vi "Antenna Comms.vi"() -> ()   [LabVIEW 2019]
panel:
  out "state":enum16{"connect", "run", "close"}(ring)
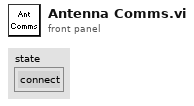
[diagram p1: front panel]
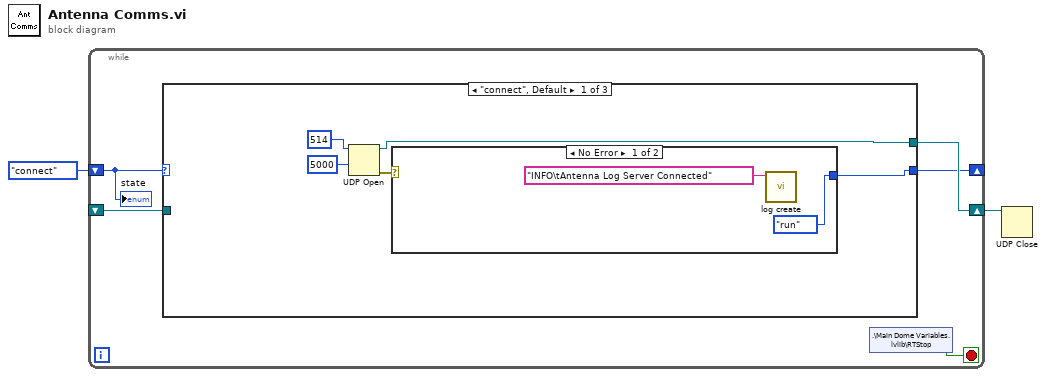
[diagram p0: block diagram]
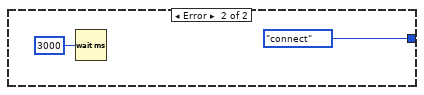
[diagram p2: hidden frame]
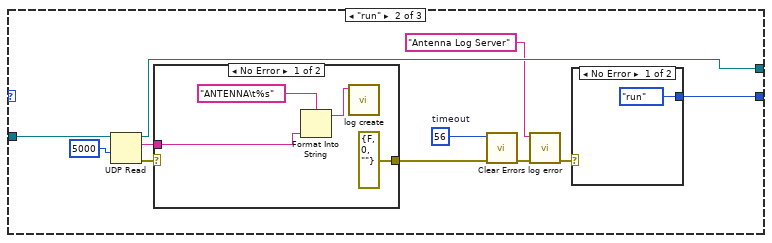
[diagram p3: hidden frame]
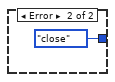
[diagram p4: hidden frame]
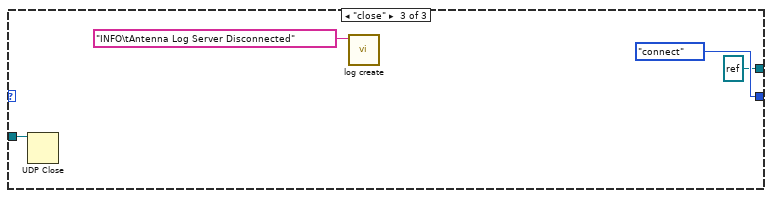
[diagram p6: hidden frame]
diagram:
  n1 = while {
    shift-right: [w3] -> _
    shift-left: enum16{"connect", "run", "close"}."connect" ("y") -> [w6]
    shift-right: [w5] -> w1
    shift-left: _ -> [w4]
    stop <- w7 stop-if-true
    n2 = case shown="\"connect\", Default" w6 {
      tunnel: [w10 w20 refnum<k16> refnum ("port")] -> w5
      tunnel: w4 -> [_ w27 w36]
      tunnel: [w8 w23 enum16{"connect", "run", "close"}."connect" ("y")] -> w3
      frame "connect", Default {
        n3 = UDP Open(9:5000 ("timeout ms (25000)"), 11:u16 514 ("port")) -> (port=w10:refnum<k16>, 0:w9:errorcluster)  [unwired: 3 in, 1 out]
        n4 = case shown="No Error" w9 {
          tunnel: [enum16{"connect", "run", "close"}."run" ("y") enum16{"connect", "run", "close"}."connect" ("y")] -> w8
          frame No Error {
            n5 = call "log create.vi"("message"="INFO\tAntenna Log Server Connected") -> ()  [unwired: 11 in]
          }
          frame Error {
            n6 = Wait (ms)(milliseconds to wait=u32 3000) -> ()  [unwired: 1 out]
          }
        }
      }
      frame "run" {
        w26 = 56  # timeout
        n7 = UDP Read(connection ID=w27, timeout ms (25000)=5000) -> (data out=w21:string, error out=w25:errorcluster, 3:w20:refnum<k16>)  [unwired: 2 in, 2 out]
        n8 = case shown="No Error" w25 {
          selector: w25 -> [_ w34]
          tunnel: [errorcluster {"status"=FALSE, "code"=0, "source"=""} ("error IO") w34] -> w24
          tunnel: w21 -> [w31 _]
          frame No Error {
            n9 = Format Into String(format string="ANTENNA\t%s", w31) -> (resulting string=w30:string)  [unwired: 2 in, 1 out]
            n10 = call "log create.vi"("message"=w30) -> ()  [unwired: 11 in]
          }
          frame Error {
          }
        }
        n11 = call <vilib>:"Clear Errors.vi"("error in (no error)"=w24, "specific error code to clear (0: all)"=w26) -> ("error out"=w19:errorcluster)  [unwired: 4 in, 1 out]
        n12 = call "log error.vi"("error in"=w19, "message"="Antenna Log Server") -> ("error out"=w17:errorcluster)  [unwired: 9 in]
        n13 = case shown="No Error" w17 {
          tunnel: [enum16{"connect", "run", "close"}."run" ("y") enum16{"connect", "run", "close"}."close" ("y")] -> w23
          frame No Error {
          }
          frame Error {
          }
        }
      }
      frame "close" {
        n14 = UDP Close(connection ID=w36) -> ()  [unwired: 1 in, 2 out]
        n15 = call "log create.vi"("message"="INFO\tAntenna Log Server Disconnected") -> ()  [unwired: 11 in]
      }
    }
    n16 = shared-variable ".\\Main Dome Variables.lvlib\\RTStop"() -> (w7:bool)  [unwired: 1 in, 1 out]
    "state" <- w6
  }
  n17 = UDP Close(connection ID=w1) -> ()  [unwired: 1 in, 2 out]
